vi "SubTest_DeleteData.vi"(8 "error in (no error)":errorcluster) -> (0 "error out":errorcluster, 1 "Deleted?T":bool)   [LabVIEW 2014, in "TableLogger_CSV_Actor.lvlib" / "TableLogger_CSV_Actor.lvclass"]
uses:
  TableLogger_CSV_Actor.lvclass
  TableLogger_Actor/TableLoggerConfig.ctl
  TableLogger_Actor/TableLoggerTypes.ctl
  TableLogger_Actor/TableLoggerBackupConfig.ctl
  TableLogger_Actor/SelectConditionCriteria.ctl
  TableLogger_SQLite_Actor/SelectConditions.ctl
  TableLogger_Actor/TableLogger_Actor.lvlib
panel:
  # "This example to check CSV Delete on Tablelogger"
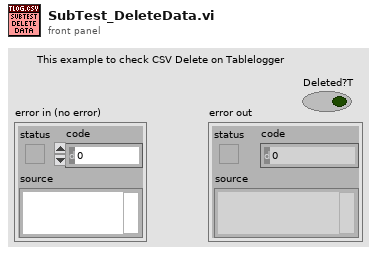
[diagram p1: front panel]
types:
  T1 = typedef "TableLogger_Actor.lvlib/SelectConditionCriteria.ctl" = cluster{"Condition Data":variant[], "Recent N.Rows":string, "Select Type":T2}
  T2 = typedef "TableLogger_Actor.lvlib/SelectConditions.ctl" = enum16{"Select All", "Select with AND Operator", "Select Most Recent Rows", "Select with OR Operator", "Select with BETWEEN Operator"}
  T3 = cluster{"Numeric Data":i32, "Float Data":dbl, "String Data":string, "Enum Data":enum16{"Enum Item 1", "Enum Item 2"}, "Array Data 2":i32[], "Cluster 2":cluster{"String":string, "Array Data 2":i32[]}, "Cluster 3":cluster{"Cluster78":cluster{"Array Data 2":i32[]}}, "Enum Data 2":enum16{"Enum Item 1", "Enum Item 2"}, "String Data 2":string, "Float Data 2":dbl, "Array Data":i32[], "Array A":cluster{"String A":string, "Array B":cluster{"String B":string, "Array B 2":cluster{"String B":string}[]}[], "Array B 2":cluster{"String B":string}[]}[]}
  T4 = cluster{"Numeric Data":i32, "Float Data":dbl, "String Data":string, "Enum Data":enum16{"Enum Item 1", "Enum Item 2"}, "Array Data 2":i32[], "Cluster 2":cluster{"String":string, "Array Data 2":i32[]}, "Cluster 3":cluster{"Cluster78":cluster{"Array Data 2":i32[]}}, "Enum Data 2":enum16{"Enum Item 1", "Enum Item 2"}, "String Data 2":string, "Float Data 2":dbl, "Array Data":i32[], "Array A":cluster{"String A":string, "Array B":cluster{"String B":string, "Array B 2":cluster{"String B":string}[]}[], "Array B 2":cluster{"String B":string}[]}[]}[]
  T5 = typedef "TableLogger_Actor.lvlib/TableLoggerConfig.ctl" = cluster{"TableLogger":T6, "DB File Path":path, "DB Backup Config":T7}
  T6 = typedef "TableLogger_Actor.lvlib/TableLoggerTypes.ctl" = enum16{"CSV Logger", "SQLite Logger"}
  T7 = typedef "TableLogger_Actor.lvlib/TableLoggerBackupConfig.ctl" = cluster{"Directory":path, "UTC Time Format":bool, "On Launch":bool, "Interval (Hours)":dbl, "Size Multiples (Bytes)":i32}
  T8 = cluster{"Numeric Data":i32, "Float Data":dbl, "String Data":string, "Enum Data":enum16{"Enum Item 1", "Enum Item 2"}}
  T9 = cluster{"Test Start Timestamp":timestamp, "Test End Timestamp":timestamp, "Test Jig Location":string, "Location Time Offset":string, "Test Jig ID":string, "Test Jig Fluid":enum16{"Liquid", "Gas"}, "Test Jig Flow":enum16{"Low", "High"}, "Control Board SN":string, "Site Number":i32, "Operator ID":string, "Operation Number":string, "DUT Serial Number":string, "DUT Product Number":string, "DUT Flow Range":i32, "DUT FW Revision":string, "DUT TP1 Offset":dbl, "DUT TP2 Offset":dbl, "DUT Cut Off1":dbl, "DUT Cut Off2":dbl, "PreCal Flow Meas":cluster{"FC Flow Set":dbl, "FM Flow Measure":dbl, "UUT Data":dbl}[], "PostCal Flow Meas":cluster{"FC Flow Set":dbl, "FM Flow Measure":dbl, "UUT Data":dbl}[], "DUT_Coeff":dbl[], "DUT_Flow_Error":dbl[], "Calibration Result":enum16{"Pass", "Fail"}}
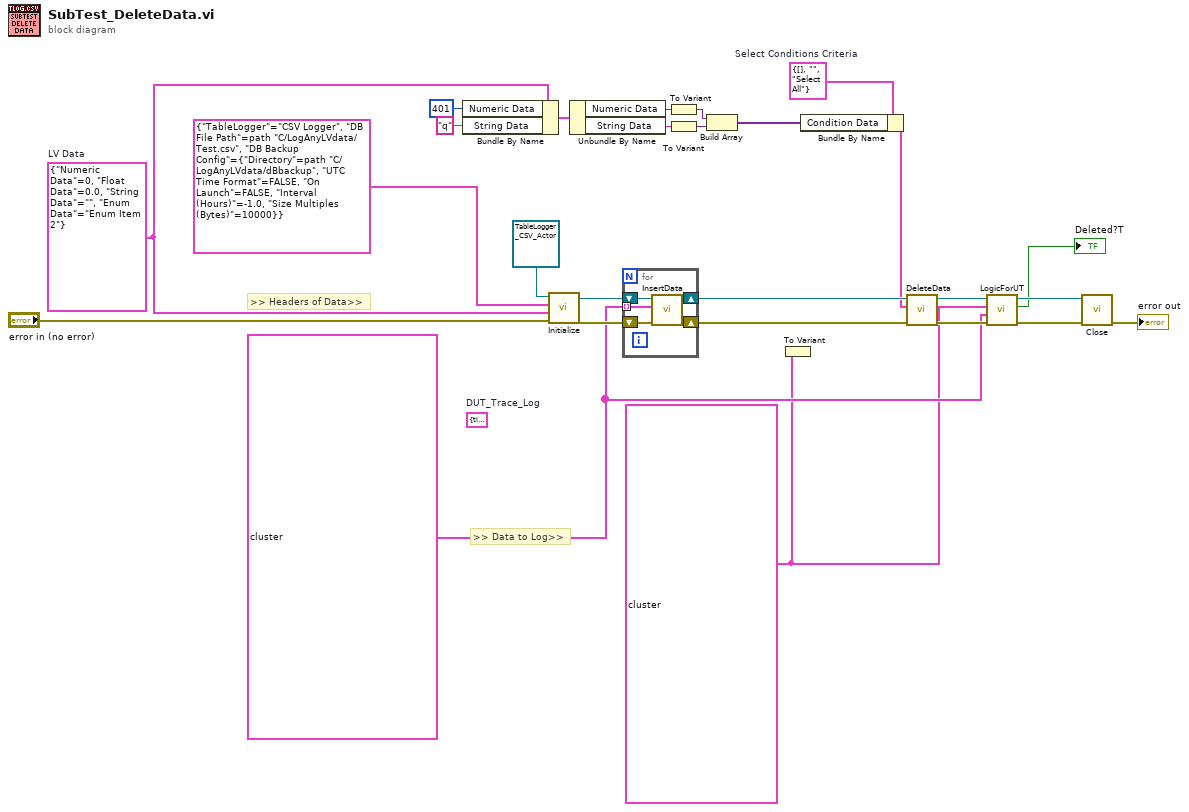
[diagram p0: block diagram]
diagram:
  w3 = T1 {"Condition Data"=[], "Recent N.Rows"="", "Select Type"=enum."Select All"}  # Select Conditions Criteria
  w12 = T3 {"Numeric Data"=987, "Float Data"=0.0, "String Data"="qwert", "Enum Data"=enum."Enum Item 2", "Array Data 2"=[0, 0, 0], "Cluster 2"={"String"="", "Array Data 2"=[0, 0, 0]}, "Cluster 3"={"Cluster78"={"Array Data 2"=[0, 0, 0]}}, "Enum Data 2"=enum."Enum Item 1", "String Data 2"="", "Float Data 2"=0.0, "Array Data"=[0, 0, 0, 4], "Array A"=[{"String A"="hello", "Array B"=[{"String B"="uq", "Array B 2"=[{"String B"="u"}, {"String B"="c"}, {"String B"="hello"}]}, {"String B"="c", "Array B 2"=[{"String B"="u"}, {"String B"="c"}, {"String B"="hello"}]}, {"String B"="hello", "Array B 2"=[{"String B"="u"}, {"String B"="c"}, {"String B"="hello"}]}], "Array B 2"=[{"String B"="u"}, {"String B"="c"}, {"String B"="hello"}]}, {"String A"="hello", "Array B"=[{"String B"="uP", "Array B 2"=[{"String B"="u"}, {"String B"="c"}, {"String B"="hello"}]}, {"String B"="c", "Array B 2"=[{"String B"="u"}, {"String B"="c"}, {"String B"="hello"}]}, {"String B"="hello", "Array B 2"=[{"String B"="u"}, {"String B"="c"}, {"String B"="hello"}]}], "Array B 2"=[{"String B"="u"}, {"String B"="c"}, {"String B"="hello"}]}]} ("LV Data")
  w13 = T4 [{"Numeric Data"=0, "Float Data"=0.0, "String Data"="", "Enum Data"=enum."Enum Item 1", "Array Data 2"=[0, 0, 0], "Cluster 2"={"String"="", "Array Data 2"=[0, 0, 0]}, "Cluster 3"={"Cluster78"={"Array Data 2"=[0, 0, 0]}}, "Enum Data 2"=enum."Enum Item 1", "String Data 2"="", "Float Data 2"=0.0, "Array Data"=[0, 0, 0, 4], "Array A"=[{"String A"="hello", "Array B"=[{"String B"="uq", "Array B 2"=[{"String B"="u"}, {"String B"="c"}, {"String B"="hello"}]}, {"String B"="c", "Array B 2"=[{"String B"="u"}, {"String B"="c"}, {"String B"="hello"}]}, {"String B"="hello", "Array B 2"=[{"String B"="u"}, {"String B"="c"}, {"String B"="hello"}]}], "Array B 2"=[{"String B"="u"}, {"String B"="c"}, {"String B"="hello"}]}, {"String A"="hello", "Array B"=[{"String B"="uP", "Array B 2"=[{"String B"="u"}, {"String B"="c"}, {"String B"="hello"}]}, {"String B"="c", "Array B 2"=[{"String B"="u"}, {"String B"="c"}, {"String B"="hello"}]}, {"String B"="hello", "Array B 2"=[{"String B"="u"}, {"String B"="c"}, {"String B"="hello"}]}], "Array B 2"=[{"String B"="u"}, {"String B"="c"}, {"String B"="hello"}]}]}, {"Numeric Data"=401, "Float Data"=0.0, "String Data"="q", "Enum Data"=enum."Enum Item 1", "Array Data 2"=[0, 0, 0], "Cluster 2"={"String"="", "Array Data 2"=[0, 0, 0]}, "Cluster 3"={"Cluster78"={"Array Data 2"=[0, 0, 0]}}, "Enum Data 2"=enum."Enum Item 1", "String Data 2"="", "Float Data 2"=0.0, "Array Data"=[0, 0, 0, 4], "Array A"=[{"String A"="hello", "Array B"=[{"String B"="uq", "Array B 2"=[{"String B"="u"}, {"String B"="c"}, {"String B"="hello"}]}, {"String B"="c", "Array B 2"=[{"String B"="u"}, {"String B"="c"}, {"String B"="hello"}]}, {"String B"="hello", "Array B 2"=[{"String B"="u"}, {"String B"="c"}, {"String B"="hello"}]}], "Array B 2"=[{"String B"="u"}, {"String B"="c"}, {"String B"="hello"}]}, {"String A"="hello", "Array B"=[{"String B"="uP", "Array B 2"=[{"String B"="u"}, {"String B"="c"}, {"String B"="hello"}]}, {"String B"="c", "Array B 2"=[{"String B"="u"}, {"String B"="c"}, {"String B"="hello"}]}, {"String B"="hello", "Array B 2"=[{"String B"="u"}, {"String B"="c"}, {"String B"="hello"}]}], "Array B 2"=[{"String B"="u"}, {"String B"="c"}, {"String B"="hello"}]}]}, {"Numeric Data"=0, "Float Data"=0.0, "String Data"="", "Enum Data"=enum."Enum Item 1", "Array Data 2"=[0, 0, 0], "Cluster 2"={"String"="", "Array Data 2"=[0, 0, 0]}, "Cluster 3"={"Cluster78"={"Array Data 2"=[0, 0, 0]}}, "Enum Data 2"=enum."Enum Item 1", "String Data 2"="", "Float Data 2"=0.0, "Array Data"=[0, 0, 0, 4], "Array A"=[{"String A"="hello", "Array B"=[{"String B"="uq", "Array B 2"=[{"String B"="u"}, {"String B"="c"}, {"String B"="hello"}]}, {"String B"="c", "Array B 2"=[{"String B"="u"}, {"String B"="c"}, {"String B"="hello"}]}, {"String B"="hello", "Array B 2"=[{"String B"="u"}, {"String B"="c"}, {"String B"="hello"}]}], "Array B 2"=[{"String B"="u"}, {"String B"="c"}, {"String B"="hello"}]}, {"String A"="hello", "Array B"=[{"String B"="uP", "Array B 2"=[{"String B"="u"}, {"String B"="c"}, {"String B"="hello"}]}, {"String B"="c", "Array B 2"=[{"String B"="u"}, {"String B"="c"}, {"String B"="hello"}]}, {"String B"="hello", "Array B 2"=[{"String B"="u"}, {"String B"="c"}, {"String B"="hello"}]}], "Array B 2"=[{"String B"="u"}, {"String B"="c"}, {"String B"="hello"}]}]}, {"Numeric Data"=0, "Float Data"=0.0, "String Data"="", "Enum Data"=enum."Enum Item 1", "Array Data 2"=[0, 0, 0], "Cluster 2"={"String"="", "Array Data 2"=[0, 0, 0]}, "Cluster 3"={"Cluster78"={"Array Data 2"=[0, 0, 0]}}, "Enum Data 2"=enum."Enum Item 1", "String Data 2"="", "Float Data 2"=0.0, "Array Data"=[0, 0, 0, 4], "Array A"=[{"String A"="hello", "Array B"=[{"String B"="uq", "Array B 2"=[{"String B"="u"}, {"String B"="c"}, {"String B"="hello"}]}, {"String B"="c", "Array B 2"=[{"String B"="u"}, {"String B"="c"}, {"String B"="hello"}]}, {"String B"="hello", "Array B 2"=[{"String B"="u"}, {"String B"="c"}, {"String B"="hello"}]}], "Array B 2"=[{"String B"="u"}, {"String B"="c"}, {"String B"="hello"}]}, {"String A"="hello", "Array B"=[{"String B"="uP", "Array B 2"=[{"String B"="u"}, {"String B"="c"}, {"String B"="hello"}]}, {"String B"="c", "Array B 2"=[{"String B"="u"}, {"String B"="c"}, {"String B"="hello"}]}, {"String B"="hello", "Array B 2"=[{"String B"="u"}, {"String B"="c"}, {"String B"="hello"}]}], "Array B 2"=[{"String B"="u"}, {"String B"="c"}, {"String B"="hello"}]}]}, {"Numeric Data"=0, "Float Data"=0.0, "String Data"="", "Enum Data"=enum."Enum Item 1", "Array Data 2"=[0, 0, 0], "Cluster 2"={"String"="", "Array Data 2"=[0, 0, 0]}, "Cluster 3"={"Cluster78"={"Array Data 2"=[0, 0, 0]}}, "Enum Data 2"=enum."Enum Item 1", "String Data 2"="", "Float Data 2"=0.0, "Array Data"=[0, 0, 0, 4], "Array A"=[{"String A"="hello", "Array B"=[{"String B"="uq", "Array B 2"=[{"String B"="u"}, {"String B"="c"}, {"String B"="hello"}]}, {"String B"="c", "Array B 2"=[{"String B"="u"}, {"String B"="c"}, {"String B"="hello"}]}, {"String B"="hello", "Array B 2"=[{"String B"="u"}, {"String B"="c"}, {"String B"="hello"}]}], "Array B 2"=[{"String B"="u"}, {"String B"="c"}, {"String B"="hello"}]}, {"String A"="hello", "Array B"=[{"String B"="uP", "Array B 2"=[{"String B"="u"}, {"String B"="c"}, {"String B"="hello"}]}, {"String B"="c", "Array B 2"=[{"String B"="u"}, {"String B"="c"}, {"String B"="hello"}]}, {"String B"="hello", "Array B 2"=[{"String B"="u"}, {"String B"="c"}, {"String B"="hello"}]}], "Array B 2"=[{"String B"="u"}, {"String B"="c"}, {"String B"="hello"}]}]}, {"Numeric Data"=0, "Float Data"=0.0, "String Data"="", "Enum Data"=enum."Enum Item 1", "Array Data 2"=[0, 0, 0], "Cluster 2"={"String"="", "Array Data 2"=[0, 0, 0]}, "Cluster 3"={"Cluster78"={"Array Data 2"=[0, 0, 0]}}, "Enum Data 2"=enum."Enum Item 1", "String Data 2"="", "Float Data 2"=0.0, "Array Data"=[0, 0, 0, 4], "Array A"=[{"String A"="hello", "Array B"=[{"String B"="uq", "Array B 2"=[{"String B"="u"}, {"String B"="c"}, {"String B"="hello"}]}, {"String B"="c", "Array B 2"=[{"String B"="u"}, {"String B"="c"}, {"String B"="hello"}]}, {"String B"="hello", "Array B 2"=[{"String B"="u"}, {"String B"="c"}, {"String B"="hello"}]}], "Array B 2"=[{"String B"="u"}, {"String B"="c"}, {"String B"="hello"}]}, {"String A"="hello", "Array B"=[{"String B"="uP", "Array B 2"=[{"String B"="u"}, {"String B"="c"}, {"String B"="hello"}]}, {"String B"="c", "Array B 2"=[{"String B"="u"}, {"String B"="c"}, {"String B"="hello"}]}, {"String B"="hello", "Array B 2"=[{"String B"="u"}, {"String B"="c"}, {"String B"="hello"}]}], "Array B 2"=[{"String B"="u"}, {"String B"="c"}, {"String B"="hello"}]}]}, {"Numeric Data"=0, "Float Data"=0.0, "String Data"="", "Enum Data"=enum."Enum Item 1", "Array Data 2"=[0, 0, 0], "Cluster 2"={"String"="", "Array Data 2"=[0, 0, 0]}, "Cluster 3"={"Cluster78"={"Array Data 2"=[0, 0, 0]}}, "Enum Data 2"=enum."Enum Item 1", "String Data 2"="", "Float Data 2"=0.0, "Array Data"=[0, 0, 0, 4], "Array A"=[{"String A"="hello", "Array B"=[{"String B"="uq", "Array B 2"=[{"String B"="u"}, {"String B"="c"}, {"String B"="hello"}]}, {"String B"="c", "Array B 2"=[{"String B"="u"}, {"String B"="c"}, {"String B"="hello"}]}, {"String B"="hello", "Array B 2"=[{"String B"="u"}, {"String B"="c"}, {"String B"="hello"}]}], "Array B 2"=[{"String B"="u"}, {"String B"="c"}, {"String B"="hello"}]}, {"String A"="hello", "Array B"=[{"String B"="uP", "Array B 2"=[{"String B"="u"}, {"String B"="c"}, {"String B"="hello"}]}, {"String B"="c", "Array B 2"=[{"String B"="u"}, {"String B"="c"}, {"String B"="hello"}]}, {"String B"="hello", "Array B 2"=[{"String B"="u"}, {"String B"="c"}, {"String B"="hello"}]}], "Array B 2"=[{"String B"="u"}, {"String B"="c"}, {"String B"="hello"}]}]}, {"Numeric Data"=0, "Float Data"=0.0, "String Data"="", "Enum Data"=enum."Enum Item 1", "Array Data 2"=[0, 0, 0], "Cluster 2"={"String"="", "Array Data 2"=[0, 0, 0]}, "Cluster 3"={"Cluster78"={"Array Data 2"=[0, 0, 0]}}, "Enum Data 2"=enum."Enum Item 1", "String Data 2"="", "Float Data 2"=0.0, "Array Data"=[0, 0, 0, 4], "Array A"=[{"String A"="hello", "Array B"=[{"String B"="uq", "Array B 2"=[{"String B"="u"}, {"String B"="c"}, {"String B"="hello"}]}, {"String B"="c", "Array B 2"=[{"String B"="u"}, {"String B"="c"}, {"String B"="hello"}]}, {"String B"="hello", "Array B 2"=[{"String B"="u"}, {"String B"="c"}, {"String B"="hello"}]}], "Array B 2"=[{"String B"="u"}, {"String B"="c"}, {"String B"="hello"}]}, {"String A"="hello", "Array B"=[{"String B"="uP", "Array B 2"=[{"String B"="u"}, {"String B"="c"}, {"String B"="hello"}]}, {"String B"="c", "Array B 2"=[{"String B"="u"}, {"String B"="c"}, {"String B"="hello"}]}, {"String B"="hello", "Array B 2"=[{"String B"="u"}, {"String B"="c"}, {"String B"="hello"}]}], "Array B 2"=[{"String B"="u"}, {"String B"="c"}, {"String B"="hello"}]}]}, {"Numeric Data"=0, "Float Data"=0.0, "String Data"="", "Enum Data"=enum."Enum Item 1", "Array Data 2"=[0, 0, 0], "Cluster 2"={"String"="", "Array Data 2"=[0, 0, 0]}, "Cluster 3"={"Cluster78"={"Array Data 2"=[0, 0, 0]}}, "Enum Data 2"=enum."Enum Item 1", "String Data 2"="", "Float Data 2"=0.0, "Array Data"=[0, 0, 0, 4], "Array A"=[{"String A"="hello", "Array B"=[{"String B"="uq", "Array B 2"=[{"String B"="u"}, {"String B"="c"}, {"String B"="hello"}]}, {"String B"="c", "Array B 2"=[{"String B"="u"}, {"String B"="c"}, {"String B"="hello"}]}, {"String B"="hello", "Array B 2"=[{"String B"="u"}, {"String B"="c"}, {"String B"="hello"}]}], "Array B 2"=[{"String B"="u"}, {"String B"="c"}, {"String B"="hello"}]}, {"String A"="hello", "Array B"=[{"String B"="uP", "Array B 2"=[{"String B"="u"}, {"String B"="c"}, {"String B"="hello"}]}, {"String B"="c", "Array B 2"=[{"String B"="u"}, {"String B"="c"}, {"String B"="hello"}]}, {"String B"="hello", "Array B 2"=[{"String B"="u"}, {"String B"="c"}, {"String B"="hello"}]}], "Array B 2"=[{"String B"="u"}, {"String B"="c"}, {"String B"="hello"}]}]}, {"Numeric Data"=0, "Float Data"=0.0, "String Data"="", "Enum Data"=enum."Enum Item 1", "Array Data 2"=[0, 0, 0], "Cluster 2"={"String"="", "Array Data 2"=[0, 0, 0]}, "Cluster 3"={"Cluster78"={"Array Data 2"=[0, 0, 0]}}, "Enum Data 2"=enum."Enum Item 1", "String Data 2"="", "Float Data 2"=0.0, "Array Data"=[0, 0, 0, 4], "Array A"=[{"String A"="hello", "Array B"=[{"String B"="uq", "Array B 2"=[{"String B"="u"}, {"String B"="c"}, {"String B"="hello"}]}, {"String B"="c", "Array B 2"=[{"String B"="u"}, {"String B"="c"}, {"String B"="hello"}]}, {"String B"="hello", "Array B 2"=[{"String B"="u"}, {"String B"="c"}, {"String B"="hello"}]}], "Array B 2"=[{"String B"="u"}, {"String B"="c"}, {"String B"="hello"}]}, {"String A"="hello", "Array B"=[{"String B"="uP", "Array B 2"=[{"String B"="u"}, {"String B"="c"}, {"String B"="hello"}]}, {"String B"="c", "Array B 2"=[{"String B"="u"}, {"String B"="c"}, {"String B"="hello"}]}, {"String B"="hello", "Array B 2"=[{"String B"="u"}, {"String B"="c"}, {"String B"="hello"}]}], "Array B 2"=[{"String B"="u"}, {"String B"="c"}, {"String B"="hello"}]}]}, {"Numeric Data"=0, "Float Data"=0.0, "String Data"="", "Enum Data"=enum."Enum Item 1", "Array Data 2"=[0, 0, 0], "Cluster 2"={"String"="", "Array Data 2"=[0, 0, 0]}, "Cluster 3"={"Cluster78"={"Array Data 2"=[0, 0, 0]}}, "Enum Data 2"=enum."Enum Item 1", "String Data 2"="", "Float Data 2"=0.0, "Array Data"=[0, 0, 0, 4], "Array A"=[{"String A"="hello", "Array B"=[{"String B"="uq", "Array B 2"=[{"String B"="u"}, {"String B"="c"}, {"String B"="hello"}]}, {"String B"="c", "Array B 2"=[{"String B"="u"}, {"String B"="c"}, {"String B"="hello"}]}, {"String B"="hello", "Array B 2"=[{"String B"="u"}, {"String B"="c"}, {"String B"="hello"}]}], "Array B 2"=[{"String B"="u"}, {"String B"="c"}, {"String B"="hello"}]}, {"String A"="hello", "Array B"=[{"String B"="uP", "Array B 2"=[{"String B"="u"}, {"String B"="c"}, {"String B"="hello"}]}, {"String B"="c", "Array B 2"=[{"String B"="u"}, {"String B"="c"}, {"String B"="hello"}]}, {"String B"="hello", "Array B 2"=[{"String B"="u"}, {"String B"="c"}, {"String B"="hello"}]}], "Array B 2"=[{"String B"="u"}, {"String B"="c"}, {"String B"="hello"}]}]}, {"Numeric Data"=401, "Float Data"=0.0, "String Data"="q", "Enum Data"=enum."Enum Item 1", "Array Data 2"=[0, 0, 0], "Cluster 2"={"String"="", "Array Data 2"=[0, 0, 0]}, "Cluster 3"={"Cluster78"={"Array Data 2"=[0, 0, 0]}}, "Enum Data 2"=enum."Enum Item 1", "String Data 2"="", "Float Data 2"=0.0, "Array Data"=[0, 0, 0, 4], "Array A"=[{"String A"="hello", "Array B"=[{"String B"="uq", "Array B 2"=[{"String B"="u"}, {"String B"="c"}, {"String B"="hello"}]}, {"String B"="c", "Array B 2"=[{"String B"="u"}, {"String B"="c"}, {"String B"="hello"}]}, {"String B"="hello", "Array B 2"=[{"String B"="u"}, {"String B"="c"}, {"String B"="hello"}]}], "Array B 2"=[{"String B"="u"}, {"String B"="c"}, {"String B"="hello"}]}, {"String A"="hello", "Array B"=[{"String B"="uP", "Array B 2"=[{"String B"="u"}, {"String B"="c"}, {"String B"="hello"}]}, {"String B"="c", "Array B 2"=[{"String B"="u"}, {"String B"="c"}, {"String B"="hello"}]}, {"String B"="hello", "Array B 2"=[{"String B"="u"}, {"String B"="c"}, {"String B"="hello"}]}], "Array B 2"=[{"String B"="u"}, {"String B"="c"}, {"String B"="hello"}]}]}]
  w4 = T8 {"Numeric Data"=0, "Float Data"=0.0, "String Data"="", "Enum Data"=enum."Enum Item 2"}  # LV Data
  (unwired) T9 {"Test Start Timestamp"=timestamp(0 s since 1904-01-01), "Test End Timestamp"=timestamp(0 s since 1904-01-01), "Test Jig Location"="asdf", "Location Time Offset"="wer", "Test Jig ID"="xcv", "Test Jig Fluid"=enum."Gas", "Test Jig Flow"=enum."High", "Control Board SN"="fgh", "Site Number"=23, "Operator ID"="op", "Operation Number"="op", "DUT Serial Number"="dt", "DUT Product Number"="dt", "DUT Flow Range"=23, "DUT FW Revision"="asdf", "DUT TP1 Offset"=24.0, "DUT TP2 Offset"=546.0, "DUT Cut Off1"=34.0, "DUT Cut Off2"=453.0, "PreCal Flow Meas"=[{"FC Flow Set"=1.0, "FM Flow Measure"=0.0, "UUT Data"=0.0}, {"FC Flow Set"=2.0, "FM Flow Measure"=0.0, "UUT Data"=0.0}, {"FC Flow Set"=3.0, "FM Flow Measure"=0.0, "UUT Data"=0.0}], "PostCal Flow Meas"=[{"FC Flow Set"=1.0, "FM Flow Measure"=0.0, "UUT Data"=0.0}, {"FC Flow Set"=2.0, "FM Flow Measure"=0.0, "UUT Data"=0.0}], "DUT_Coeff"=[1.0, 2.0], "DUT_Flow_Error"=[1.0, 2.0], "Calibration Result"=enum."Fail"}  # DUT_Trace_Log
  # ">> Headers of Data>>"
  # ">> Data to Log>>"
  n1 = Bundle By Name(cluster=w4, "Numeric Data"=401, "String Data"="q") -> (w9:T8)
  n2 = call-dynamic "Initialize.vi"("error in (no error)"="error in (no error)", "Data Cluster (for Headers)"=w4, "TableLogger Config"=T5 {"TableLogger"=enum."CSV Logger", "DB File Path"=path "C:/LogAnyLVdata/Test.csv", "DB Backup Config"={"Directory"=path "C:/LogAnyLVdata/dBbackup", "UTC Time Format"=FALSE, "On Launch"=FALSE, "Interval (Hours)"=-1.0, "Size Multiples (Bytes)"=10000}}, "object in"=refnum<class "TableLogger_CSV_Actor.lvclass"> refnum) -> ("error out"=w24:errorcluster, "object out"=w25:refnum<class "TableLogger_CSV_Actor.lvclass">)  [unwired: 6 in]
  n3 = Unbundle By Name(w9) -> ("Numeric Data"=w7:i32, "String Data"=w8:string)
  n4 = for {
    shift-right: [w28] -> w19
    shift-left: w25 -> [w30]
    shift-right: [w27] -> w20
    shift-left: w24 -> [w29]
    tunnel: w13 -> [w26] mode=indexing
    n5 = call-dynamic "InsertData.vi"("error in (no error)"=w29, "Data Cluster"=w26, "object in"=w30) -> ("error out"=w27:errorcluster, "object out"=w28:refnum<class "TableLogger_CSV_Actor.lvclass">)  [unwired: 7 in]
  }
  n6 = To Variant(anything=w7) -> (Variant=w6:variant)
  n7 = To Variant(anything=w8) -> (Variant=w5:variant)
  n8 = Build Array(w6, w5) -> (w2:variant[])
  n9 = To Variant(anything=w12) -> ()  [unwired: 1 out]
  n10 = Bundle By Name(cluster=w3, "Condition Data"=w2) -> (w1:T1)
  n11 = call-dynamic "DeleteData.vi"("error in (no error)"=w20, "Select Conditions Criteria"=w1, "object in"=w19) -> ("error out"=w16:errorcluster, "object out"=w17:refnum<class "TableLogger_CSV_Actor.lvclass">)  [unwired: 6 in, 1 out]
  n12 = call "LogicForUT.vi"("error in (no error)"=w16, "Array"=w13, "LV Data"=w12, "TableLogger_CSV_Actor in"=w17) -> ("error out"=w14:errorcluster, "Deleted?T"=→"Deleted?T":bool)  [unwired: 4 in, 2 out]
  n13 = call-dynamic "Close.vi"("error in (no error)"=w14, "object in"=w17) -> ("error out"=→"error out":errorcluster)  [unwired: 8 in, 1 out]
